vi "Tree Control.vi"() -> ()   [LabVIEW 2021, in "Tree Map.lvlib"]
doc: "<b>Author:</b> Piotr Kruczkowski <PrimaryKey>\n<b>License:</b> NewBSD\n\nCopyright (c) 2019, National Instruments\nAll rights reserved.\n\nRedistribution and use in source and binary forms, with or without\nmodification, are permitted provided that the following conditions are met:\n1. Redistributions of source code must retain the above copyright\n notice, this list of conditions and the following disclaimer.\n2. Redistributions in binary form must reproduce the above copyright\n notice, this list of conditions and the following disclaimer in the\n documentation and/or other materials provided with the distribution.\n3. Neither the name of National Instruments nor the\n names of its contributors may be used to endorse or promote products\n derived from this software without specific prior written permission.\n\nTHIS SOFTWARE IS PROVIDED BY National Instruments ''AS IS'' AND ANY\nEXPRESS OR IMPLIED WARRANTIES, INCLUDING, BUT NOT LIMITED TO, THE IMPLIED\nWARRANTIES OF MERCHANTABILITY AND FITNESS FOR A PARTICULAR PURPOSE ARE\nDISCLAIMED. IN NO EVENT SHALL National Instruments BE LIABLE FOR ANY\nDIRECT, INDIRECT, INCIDENTAL, SPECIAL, EXEMPLARY, OR CONSEQUENTIAL DAMAGES\n(INCLUDING, BUT NOT LIMITED TO, PROCUREMENT OF SUBSTITUTE GOODS OR SERVICES;\nLOSS OF USE, DATA, OR PROFITS; OR BUSINESS INTERRUPTION) HOWEVER CAUSED AND\nON ANY THEORY OF LIABILITY, WHETHER IN CONTRACT, STRICT LIABILITY, OR TORT\n(INCLUDING NEGLIGENCE OR OTHERWISE) ARISING IN ANY WAY OUT OF THE USE OF THIS\nSOFTWARE, EVEN IF ADVISED OF THE POSSIBILITY OF SUCH DAMAGE."
uses:
  <vilib>/National Instruments/Tree Map/Tree Map.lvlib
  <vilib>/National Instruments/Tree Map/API/List Roots.vi
  <vilib>/National Instruments/Tree Map/Utility/Into Tree Control Items.vi
panel:
  out "Tree Control Items":T1(array[cluster])
  out "Node Data":T2={"Child Paths Set"={}, "Name"="MySubNode", "Data"="0.68", "Attributes"={}}
  out "Node Path":string="\\Root\\MyNode\\MySubNode"
  in  "Tree Control - Click on the elements":string(tree)="\\Root\\MyNode\\MySubNode"
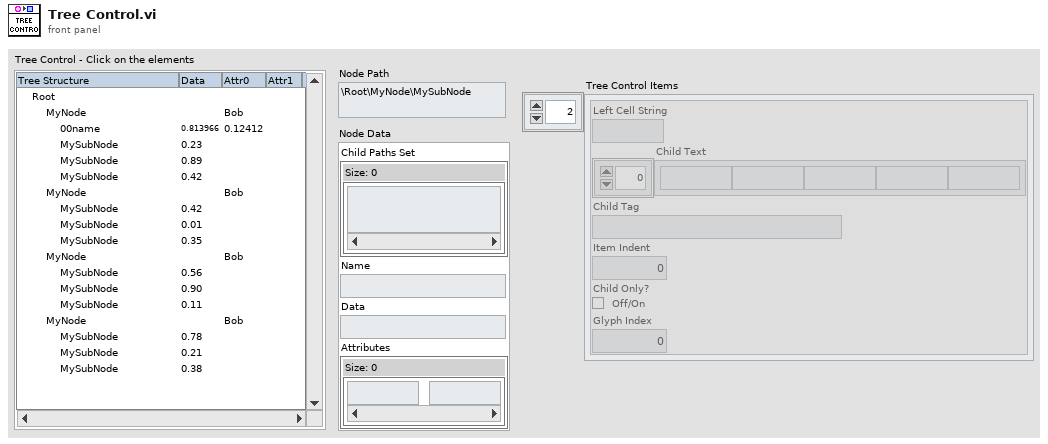
[diagram p1: front panel]
types:
  T1 = cluster{"Left Cell String":string, "Child Text":string[], "Child Tag":string, "Item Indent":i32, "Child Only?":bool, "Glyph Index":i32}[]
  T2 = cluster{"Child Paths Set":set{string}, "Name":string, "Data":string, "Attributes":map{string, string}}
  T3 = typedef "Tree Map.lvlib/Tree Map Data.ctl" = map{string, cluster{"Child Paths Set":set{string}, "Name":string, "Data":string, "Attributes":map{string, string}}}
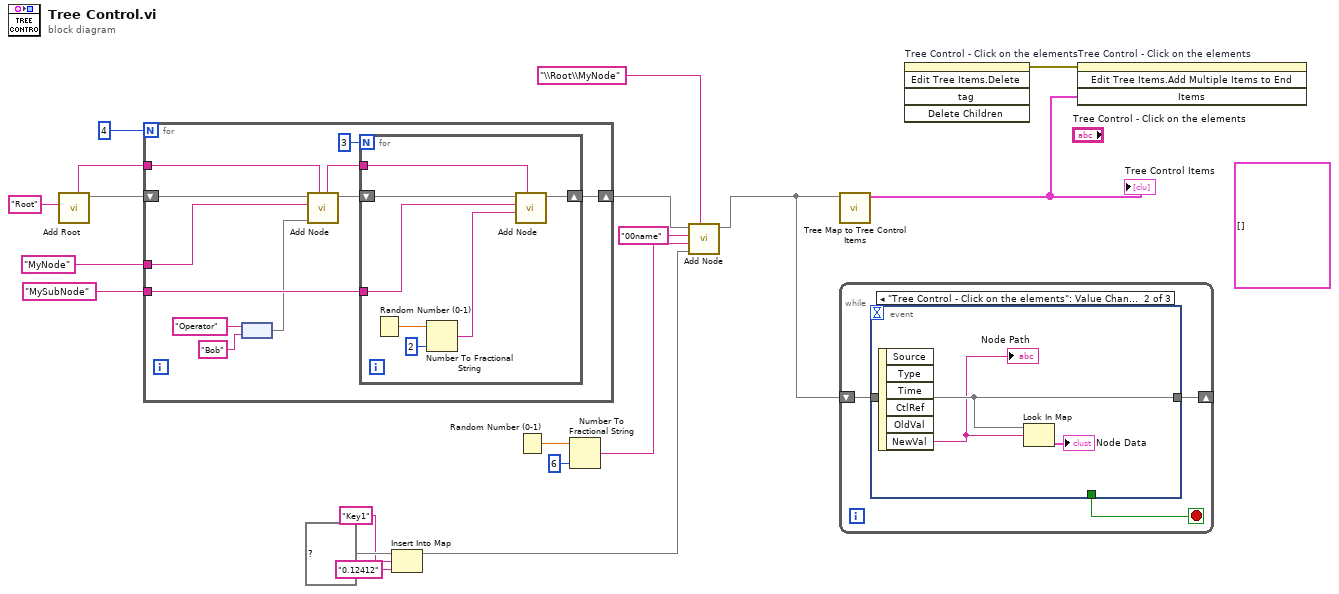
[diagram p0: block diagram]
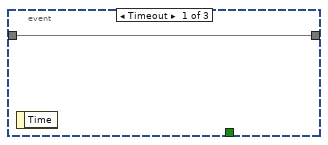
[diagram p2: hidden frame]
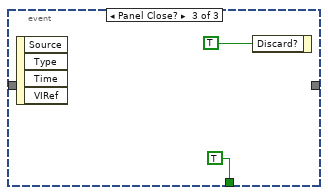
[diagram p3: hidden frame]
diagram:
  (unwired) T1 [] ("Tree Control Items")
  n1 = call <vilib>:"Add Root.vi"("New Root Name"="Root") -> ("Tree Map Out"=w19:T3, "Root Path"=w18:string)  [unwired: 9 in]
  n2 = for {
    N: 4 -> [_]
    tunnel: w18 -> [w29]
    tunnel: "MyNode" ("New Node Name") -> [w28]
    shift-right: [w27] -> w11
    shift-left: w19 -> [w30]
    tunnel: "MySubNode" ("New Node Name") -> [w24]
    n3 = node("Operator" ("key"), "Bob" ("key")) -> (w20:map{string, string})
    n4 = call <vilib>:"Add Node.vi"("Parent Path"=w29, "Attributes"=w20, "New Node Name"=w28, "Tree Map In"=w30) -> ("Tree Map Out"=w26:T3, "New Node Path"=w25:string)  [unwired: 5 in, 1 out]
    n5 = for {
      N: 3 -> [_]
      shift-right: [w36] -> w27
      shift-left: w26 -> [w37]
      tunnel: w25 -> [w35]
      tunnel: w24 -> [w34]
      n6 = Random Number (0-1)() -> (number: 0 to 1=w33:dbl)
      n7 = Number To Fractional String(number=w33, precision (6)=i16 2) -> (F-format string=w31:string)  [unwired: 2 in]
      n8 = call <vilib>:"Add Node.vi"("Parent Path"=w35, "Data"=w31, "New Node Name"=w34, "Tree Map In"=w37) -> ("Tree Map Out"=w36:T3)  [unwired: 5 in, 2 out]
    }
  }
  n9 = Insert Into Map(map in=map{string, string} {} ("Attributes"), key="Key1", value="0.12412") -> (map out=w3:map{string, string})  [unwired: 2 out]
  n10 = Random Number (0-1)() -> (number: 0 to 1=w6:dbl)
  n11 = Number To Fractional String(number=w6, precision (6)=i16 6) -> (F-format string=w5:string)  [unwired: 2 in]
  n12 = call <vilib>:"Add Node.vi"("Parent Path"="\\Root\\MyNode", "Attributes"=w3, "Data"=w5, "New Node Name"="00name", "Tree Map In"=w11) -> ("Tree Map Out"=w10:T3)  [unwired: 4 in, 2 out]
  n13 = call <vilib>:"Tree Map to Tree Control Items.vi"("Tree Map In"=w10) -> ("Tree Control Items"=w12:T1)  [unwired: 10 in]
  "Tree Control Items" <- w12
  n14 = while {
    shift-right: [w40] -> _
    shift-left: w10 -> [w39]
    stop <- w38 stop-if-true
    n15 = event shown="[1] \"Tree Control - Click on the elements\": Value Change" {
      selector: _ -> [_ _ _]
      dyn-events: _ -> [_ _ _]
      timeout: _ -> [_ _ _]
      tunnel: [w41 w44 _] -> w40
      tunnel: w39 -> [w41 w44 _]
      tunnel: [_ _ TRUE ("Discard?")] -> w38
      event Timeout {
        n16 = event-data() -> ()  [unwired: 1 in, 1 out]
      }
      event "Tree Control - Click on the elements": Value Change {
        n17 = event-data() -> ("NewVal"=w42:string)  [unwired: 1 in, 5 out]
        "Node Path" <- w42
        n18 = Look In Map(map=w44, key=w42) -> (value=→"Node Data":T2)  [unwired: 1 in, 1 out]
      }
      event Panel Close? {
        n19 = event-data() -> ()  [unwired: 1 in, 4 out]
        n20 = event-data("Discard?"=TRUE) -> ()  [unwired: 1 in, 1 out]
      }
    }
  }
  n21 = invoke on="Tree Control - Click on the elements" class="Tree (strict)" method="Edit Tree Items.Delete"() -> (error out=w16:errorcluster)  [unwired: 5 in, 4 out]
  n22 = invoke on="Tree Control - Click on the elements" class="Tree (strict)" method="Edit Tree Items.Add Multiple Items to End"(error in=w16, "Items"=w12) -> ()  [unwired: 2 in, 4 out]
